vi "Make Transfer Log.vi"() -> ()   [LabVIEW 2020]
uses:
  Orca Data Spooler Type Defs/Orca Data Spooler Transfer Log Type.ctl
panel:
  out "Selected Path":path caption="selected path"
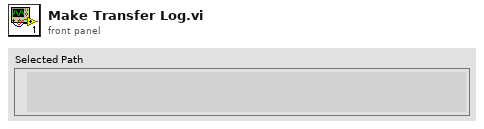
[diagram p1: front panel]
types:
  T1 = typedef "Orca Data Spooler Transfer Log Type.ctl" = cluster{"File Name":string, "Status":string}
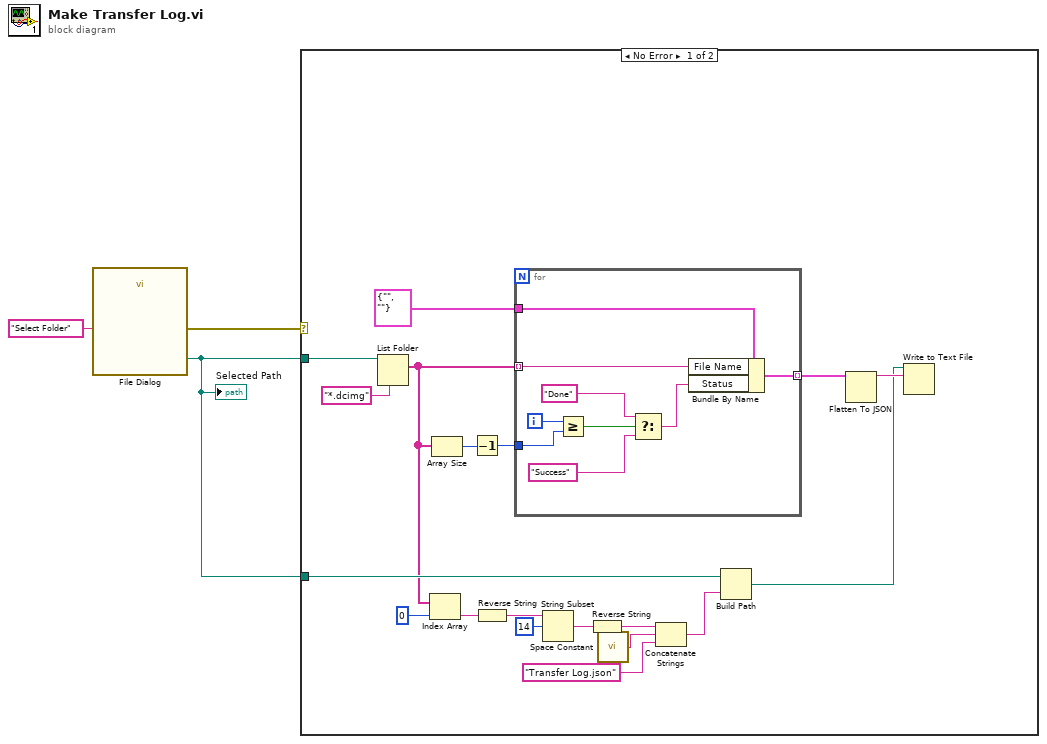
[diagram p0: block diagram]
diagram:
  n1 = call "File Dialog"("prompt"="Select Folder") -> ("selected path"=w1:path, "error out"=w2:errorcluster)  [unwired: 11 in, 2 out]
  "Selected Path" <- w1
  n2 = case shown="No Error" w2 {
    tunnel: w1 -> [w22 _]
    tunnel: w1 -> [w15 _]
    frame No Error {
      n3 = List Folder(path=w22, pattern="*.dcimg") -> (filenames=w13:string[])  [unwired: 2 in, 3 out]
      n4 = Index Array(array=w13, index=0) -> (element=w11:string)
      n5 = Array Size(array=w13) -> (size(s)=w19:i32)
      n6 = Decrement(x=w19) -> (x-1=w18:i32)
      n7 = Reverse String(1:w11) -> (0:w10:string)
      n8 = for {
        tunnel: w13 -> [w30] mode=indexing
        tunnel: T1 {"File Name"="", "Status"=""} ("Transfer Log Type") -> [w31]
        tunnel: [w23] -> w17 mode=indexing
        tunnel: w18 -> [w28]
        i -> [w29]
        n9 = Greater Or Equal?(x=w29, y=w28) -> (x >= y?=w27:bool)
        n10 = Select(t="Done", s=w27, f="Success") -> (s? t:f=w24:string)
        n11 = Bundle By Name(cluster=w31, "File Name"=w30, "Status"=w24) -> (w23:T1)
      }
      n12 = String Subset(string=w10, offset (0)=14) -> (substring=w8:string)  [unwired: 1 in]
      n13 = Reverse String(1:w8) -> (0:w7:string)
      n14 = call <vilib>:"Space Constant.vi"() -> ("String"=w6:string)
      n15 = Concatenate Strings(w7, w6, "Transfer Log.json") -> (w4:string)
      n16 = Build Path(base path=w15, name or relative path=w4) -> (appended path=w14:path)
      n17 = Flatten To JSON(anything=w17) -> (JSON string=w16:string)  [unwired: 2 in, 1 out]
      n18 = Write to Text File(file (use dialog)=w14, text=w16) -> ()  [unwired: 2 in, 3 out]
    }
    frame Error {
    }
  }
